vi "OPC UA Server.vi"() -> ()   [LabVIEW 2019]
uses:
  <vilib>/OPCUA/controls/Data Type.ctl
  <vilib>/OPCUA/NI OPC UA Server.lvlib
panel:
  in  "stop":bool
  out "Item path temp C":string
  out "Server endpoint URL":string
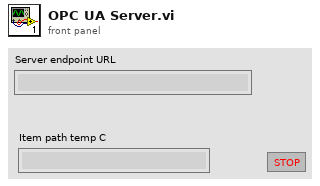
[diagram p1: front panel]
types:
  T1 = typedef "Data Type.ctl" = u16
  T2 = cluster{"name":string, "data type":T1, "access level":u16, "description":string}
  T3 = typedef "OPC UA Server Refnum.ctl" = refnum<k21>
  T4 = typedef "NodeId.ctl" = string
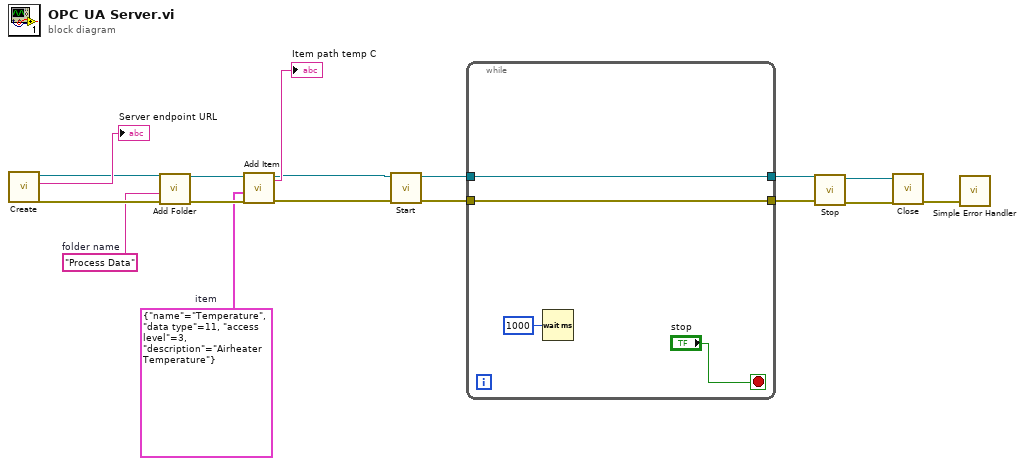
[diagram p0: block diagram]
diagram:
  w11 = T2 {"name"="Temperature", "data type"=11, "access level"=3, "description"="Airheater Temperature"}  # item
  w14 = "Process Data"  # folder name
  n1 = call <vilib>:"Create.vi"() -> ("error out"=w16:errorcluster, "server endpoint URL"=→"Server endpoint URL":string, "OPC UA server refnum out"=w15:T3)  [unwired: 9 in]
  n2 = call <vilib>:"Add Folder.vi"("error in (no error)"=w16, "folder name"=w14, "OPC UA server refnum in"=w15) -> ("error out"=w12:errorcluster, "OPC UA server refnum out"=w13:T3)  [unwired: 5 in, 1 out]
  n3 = call <vilib>:"Add Item.vi"("error in (no error)"=w12, "item"=w11, "OPC UA server refnum in"=w13) -> ("error out"=w1:errorcluster, "item node ID"=→"Item path temp C":T4, "OPC UA server refnum out"=w2:T3)  [unwired: 4 in, 1 out]
  n4 = call <vilib>:"Start.vi"("error in (no error)"=w1, "OPC UA server refnum in"=w2) -> ("error out"=w9:errorcluster, "OPC UA server refnum out"=w10:T3)  [unwired: 7 in, 1 out]
  n5 = while {
    tunnel: w10 -> [w19]
    tunnel: w9 -> [w18]
    tunnel: [w19] -> w8
    tunnel: [w18] -> w7
    stop <- "stop" stop-if-true
    n6 = Wait (ms)(milliseconds to wait=u32 1000) -> ()  [unwired: 1 out]
  }
  n7 = call <vilib>:"Stop.vi"("error in (no error)"=w7, "OPC UA server refnum in"=w8) -> ("error out"=w5:errorcluster, "OPC UA server refnum out"=w6:T3)  [unwired: 8 in]
  n8 = call <vilib>:"Close.vi"("error in (no error)"=w5, "OPC UA server refnum in"=w6) -> ("error out"=w4:errorcluster)  [unwired: 9 in]
  n9 = call <vilib>:"Simple Error Handler.vi"("error in (no error)"=w4) -> ()  [unwired: 4 in, 5 out]
